vi "0x字符串转换正常显示.vi"(1 "普通字符串":string) -> (15 "0x普通字符串":string)   [LabVIEW 2019]
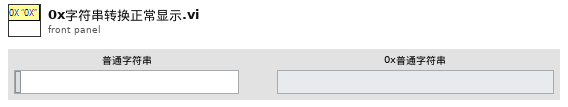
[diagram p1: front panel]
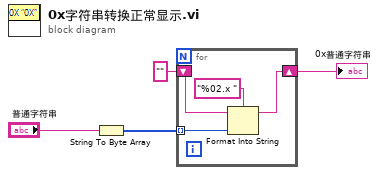
[diagram p0: block diagram]
diagram:
  n1 = String To Byte Array(string="普通字符串") -> (unsigned byte array=w3:u8[])
  n2 = for {
    tunnel: w3 -> [w7] mode=indexing
    shift-right: [w5] -> w2
    shift-left: "" -> [w6]
    n3 = Format Into String(format string="%02.x " ("格式字符串"), initial string=w6, w7) -> (resulting string=w5:string)  [unwired: 1 in, 1 out]
  }
  "0x普通字符串" <- w2
